vi "Configure Hardware.vi"(8 "error in (no error)":errorcluster caption="错误输入（无错误）", 11 "Hardware Resources in":T1={"PLC设置"={"端口选择"="COM3", "波特率"=0, "校检"=0, "数据位"=0}, "动作设置"={"自动跳法测试动作"={"夹紧"={"PLC指令"={"变量类型"=2, "PLC地址"="0", "16位/32位"=0, "写入数据(写入时有效)"=""}}, "分中"={}, "通油"={"打开主阀"={"变量类型"=2, "PLC地址"="0", "16位/32位"=0, "写入数据(写入时有效)"=""}, "打开电磁阀"={"变量类型"=2, "PLC地址"="0", "16位/32位"=0, "写入数据(写入时有效)"=""}}, "自动对中"={}, "内泄漏测试"={}, "压销"={"PLC指令"={"变量类型"=2, "PLC地址"="0", "16位/32位"=0, "写入数据(写入时有效)"=""}}}}} caption="硬件资源输入" {"动作设置"."自动跳法测试动作"."压销"."PLC指令"."16位/32位" items=["16bit", "32bit"]; "动作设置"."自动跳法测试动作"."压销"."PLC指令"."变量类型" items=["X", "Y", "M", "D"]; "动作设置"."自动跳法测试动作"."通油"."打开电磁阀"."16位/32位" items=["16bit", "32bit"]; "动作设置"."自动跳法测试动作"."通油"."打开电磁阀"."变量类型" items=["X", "Y", "M", "D"]; "动作设置"."自动跳法测试动作"."通油"."打开主阀"."16位/32位" items=["16bit", "32bit"]; "动作设置"."自动跳法测试动作"."通油"."打开主阀"."变量类型" items=["X", "Y", "M", "D"]; "动作设置"."自动跳法测试动作"."夹紧"."PLC指令"."16位/32位" items=["16bit", "32bit"]; "动作设置"."自动跳法测试动作"."夹紧"."PLC指令"."变量类型" items=["X", "Y", "M", "D"]; "PLC设置"."数据位" items=["7"=7, "8"=8]; "PLC设置"."校检" items=["无", "偶", "奇"]; "PLC设置"."波特率" items=["9600"=9600, "19200"=19200, "115200"=115200]}) -> (0 "error out":errorcluster caption="错误输出", 3 "Hardware Resources out":T1={"PLC设置"={"端口选择"="COM3", "波特率"=0, "校检"=0, "数据位"=0}, "动作设置"={"自动跳法测试动作"={"夹紧"={"PLC指令"={"变量类型"=2, "PLC地址"="0", "16位/32位"=0, "写入数据(写入时有效)"=""}}, "分中"={}, "通油"={"打开主阀"={"变量类型"=2, "PLC地址"="0", "16位/32位"=0, "写入数据(写入时有效)"=""}, "打开电磁阀"={"变量类型"=2, "PLC地址"="0", "16位/32位"=0, "写入数据(写入时有效)"=""}}, "自动对中"={}, "内泄漏测试"={}, "压销"={"PLC指令"={"变量类型"=2, "PLC地址"="0", "16位/32位"=0, "写入数据(写入时有效)"=""}}}}} caption="硬件资源输出" {"动作设置"."自动跳法测试动作"."压销"."PLC指令"."16位/32位" items=["16bit", "32bit"]; "动作设置"."自动跳法测试动作"."压销"."PLC指令"."变量类型" items=["X", "Y", "M", "D"]; "动作设置"."自动跳法测试动作"."通油"."打开电磁阀"."16位/32位" items=["16bit", "32bit"]; "动作设置"."自动跳法测试动作"."通油"."打开电磁阀"."变量类型" items=["X", "Y", "M", "D"]; "动作设置"."自动跳法测试动作"."通油"."打开主阀"."16位/32位" items=["16bit", "32bit"]; "动作设置"."自动跳法测试动作"."通油"."打开主阀"."变量类型" items=["X", "Y", "M", "D"]; "动作设置"."自动跳法测试动作"."夹紧"."PLC指令"."16位/32位" items=["16bit", "32bit"]; "动作设置"."自动跳法测试动作"."夹紧"."PLC指令"."变量类型" items=["X", "Y", "M", "D"]; "PLC设置"."数据位" items=["7"=7, "8"=8]; "PLC设置"."校检" items=["无", "偶", "奇"]; "PLC设置"."波特率" items=["9600"=9600, "19200"=19200, "115200"=115200]})   [LabVIEW 2015, in "Action.lvlib"]
doc: "配置硬件。"
uses:
  Action.lvlib
  <vilib>/DAQmx/create/channels.llb/DAQmx Create Channel (AI-Voltage-Basic).vi
  <vilib>/DAQmx/configure/timing.llb/DAQmx Timing (Sample Clock).vi
  Hardware Configuration.ctl
  PLC/PLC.lvlib
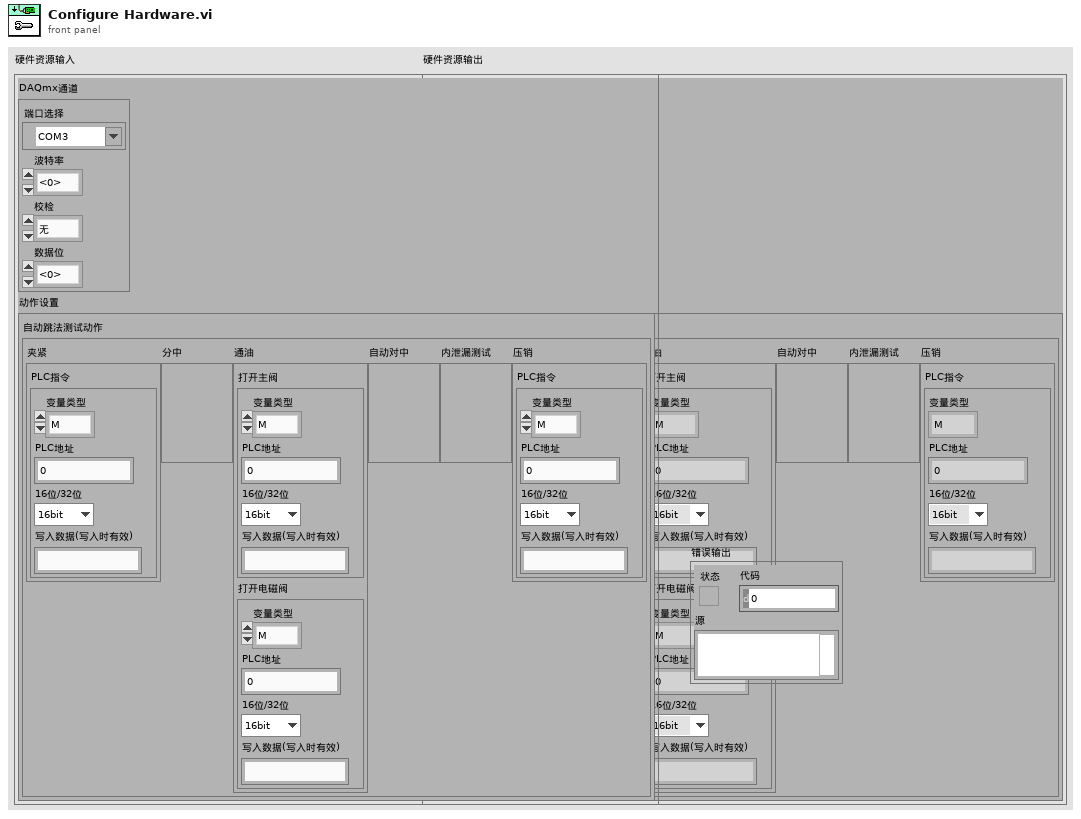
[diagram p1: front panel]
types:
  T1 = typedef "Action.lvlib/Hardware Configuration.ctl" = cluster{"PLC设置":T2, "动作设置":T3}
  T2 = typedef "PLC.lvlib/PLC设置.ctl" = cluster{"端口选择":refnum<visa-resource-name>, "波特率":u32, "校检":u32, "数据位":u32}
  T3 = typedef "Action.lvlib/动作设置.ctl" = cluster{"自动跳法测试动作":T4}
  T4 = typedef "Action.lvlib/自动调阀测试动作设置.ctl" = cluster{"夹紧":cluster{"PLC指令":T5}, "分中":cluster{}, "通油":cluster{"打开主阀":T5, "打开电磁阀":T5}, "自动对中":cluster{}, "内泄漏测试":cluster{}, "压销":cluster{"PLC指令":T5}}
  T5 = typedef "PLC.lvlib/PLC指令.ctl" = cluster{"变量类型":u32, "PLC地址":string, "16位/32位":u32, "写入数据(写入时有效)":string}
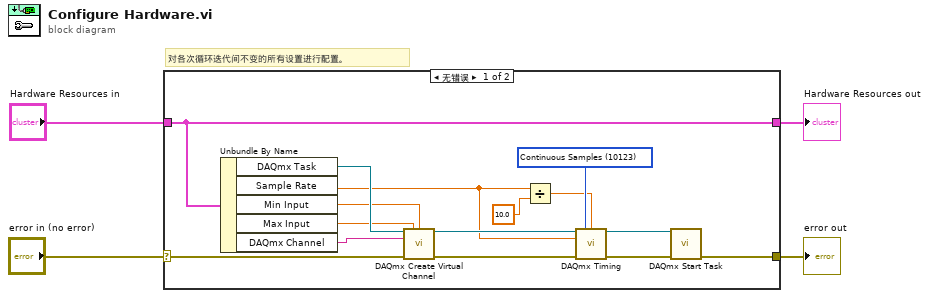
[diagram p0: block diagram]
diagram:
  # "对各次循环迭代间不变的所有设置进行配置。"
  n1 = case shown="无错误" "error in (no error)" {
    selector: "error in (no error)" -> [w13 w20]
    tunnel: [w5 w20] -> w3
    tunnel: "Hardware Resources in" -> [w12 w21]
    tunnel: [w12 w21] -> w1
    frame No Error {
      w11 = 10123 items=["Finite Samples"=10178, "Continuous Samples"=10123, "Hardware Timed Single Point"=12522] ("sample mode")
      n2 = Unbundle By Name(w12) -> ("DAQmx Task"=w19:refnum<k21>, "Sample Rate"=w10:dbl, "Min Input"=w16:dbl, "Max Input"=w17:dbl, "DAQmx Channel"=w18:tag)
      n3 = call-poly <vilib>:"DAQmx Create Virtual Channel.vi"("task in"=w19, "maximum value"=w17, "minimum value"=w16, "physical channels"=w18, "error in"=w13) -> ("task out"=w15:refnum<k21>, "error out"=w14:errorcluster)  [unwired: 9 in]
      n4 = Divide(x=w10, y=10.0) -> (x/y=w8:dbl)
      n5 = call-poly <vilib>:"DAQmx Timing.vi"("task/channels in"=w15, "sample mode"=w11, "samples per channel"=w8, "rate"=w10, "error in"=w14) -> ("task out"=w6:refnum<k21>, "error out"=w7:errorcluster)  [unwired: 9 in]
      n6 = call <vilib>:"DAQmx Start Task.vi"("task/channels in"=w6, "error in"=w7) -> ("error out"=w5:errorcluster)  [unwired: 12 in, 1 out]
    }
    frame Error {
    }
  }
  "Hardware Resources out" <- w1
  "error out" <- w3
